vi "Three Button Dialog CORE - JKI.vi"(4 "Allow user to close window? (TRUE)":bool=TRUE, 5 "Justify Message (Left)":enum16{"Left", "Center", "Right"}(ring), 6 "Keyboard Shortcuts (Left is <Enter>)":T2={"Left Button Key Shortcut"={"Control"=FALSE, "Shift"=FALSE, "Key"="<Enter>"}, "Center Button Key Shortcut"={"Control"=FALSE, "Shift"=FALSE, "Key"=""}, "Right Button Key Shortcut"={"Control"=FALSE, "Shift"=FALSE, "Key"=""}}, 7 "Window Title (\"\")":string, 8 "Right Button Text (\"Cancel\")":string="Cancel", 9 "Center Button Text (\"No\")":string="No", 10 "Left Button Text (\"Yes\")":string="Yes", 11 "message":string) -> (3 "Which Button?":T1(ring)=enum."Center Button")   [LabVIEW 2013]
doc: "This is an example to show how someone can use the JKI State Machine. We show how you can refactor existing code. We have taken the 3 button dialog that ships with the base version of LabVIEW and upgraded it to use the JKI State Machine template.\n<B>The original VI is located at: <vi.lib>\\Utility\\error.llb\\Three Button Dialog CORE.vi</B>\n\nFor instructions on how to use the JKI State Machine, examples and video tutorials, visit:\nhttp://jkisoft.com/state-machine/\n\nJKI State Machine™ Example Code\nhttp://jkisoft.com/state-machine/\nCopyright (C) 2005-2008, JKI <info@jkisoft.com>\nALL RIGHTS RESERVED"
panel:
  in  "Right Button":bool
  in  "Center Button":bool
  in  "Left Button":bool
  out "C-Message":string
  in  "OK":string="OK"
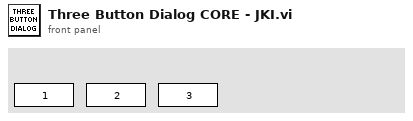
[diagram p1: front panel]
types:
  T1 = enum16{"Left Button", "Center Button", "Right Button", "Window Close"}
  T2 = cluster{"Left Button Key Shortcut":cluster{"Control":bool, "Shift":bool, "Key":string}, "Center Button Key Shortcut":cluster{"Control":bool, "Shift":bool, "Key":string}, "Right Button Key Shortcut":cluster{"Control":bool, "Shift":bool, "Key":string}}
  T3 = enum32{"invalid app kind", "Development System", "Run Time System", "Student Edition", "Embedded LabVIEW", "Evaluation", "Custom"}
  T4 = enum32{"Invalid", "Standard", "Closed", "Hidden", "Minimized", "Maximized"}
  T5 = cluster{"left":i16, "top":i16, "right":i16, "bottom":i16}
  T6 = cluster{"Core":cluster{"Current VI Reference":refnum<vi>, "Close Panel on Exit?":bool}, "Justify Message (Left)":enum16{"Left", "Center", "Right"}, "Allow user to close window? (TRUE)":bool, "Keyboard Shortcuts (Left is <Enter>)":cluster{"Left Button Key Shortcut":cluster{"Control":bool, "Shift":bool, "Key":string}, "Center Button Key Shortcut":cluster{"Control":bool, "Shift":bool, "Key":string}, "Right Button Key Shortcut":cluster{"Control":bool, "Shift":bool, "Key":string}}, "Left Button Text (\"Yes\")":string, "Center Button Text (\"No\")":string, "Right Button Text (\"Cancel\")":string, "message":string, "OK":string, "Left Visible?":bool, "Center Visible?":bool, "Right Visible?":bool, "C Message Height":u32, "minimum width for message":i32, "mimimum window width":i32, "minimum window width for buttons":i32, "Left Button Position:Left":i32, "grid spacing":i32, "grid spacing X2":i32, "window center":i32, "Window Title (\"\")":string, "Original FP.Title":string, "Which Button?":enum16{"Left Button", "Center Button", "Right Button", "Window Close"}}
  T7 = cluster{"Current VI Reference":refnum<vi>, "Close Panel on Exit?":bool}
  T8 = cluster{"Control":bool, "Shift":bool, "Key":string}
  T9 = cluster{bool, "Control":bool, "Shift":bool, "Key":string}
  T10 = typedef "LVRectTypeDef.ctl" = cluster{"Left":i16, "Top":i16, "Right":i16, "Bottom":i16}
  T11 = typedef "LVPointTypeDef.ctl" = cluster{"Horizontal":i16, "Vertical":i16}
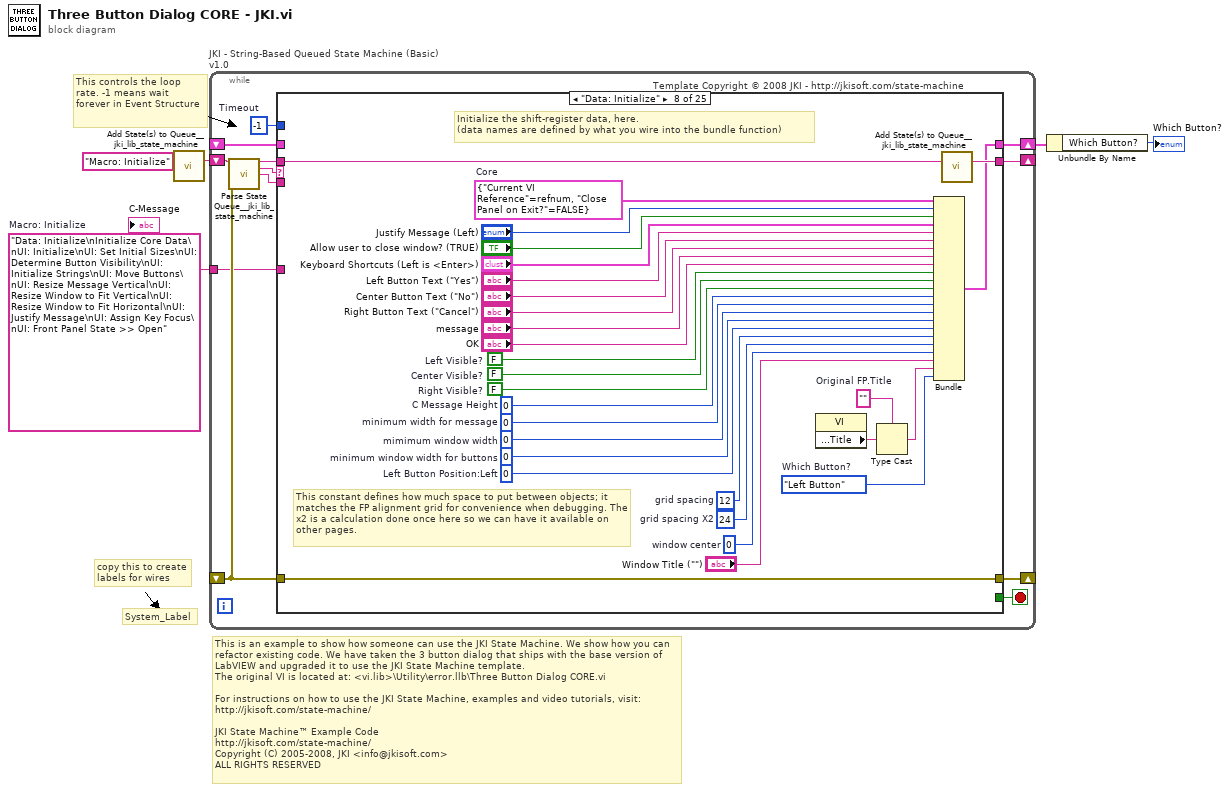
[diagram p0: block diagram]
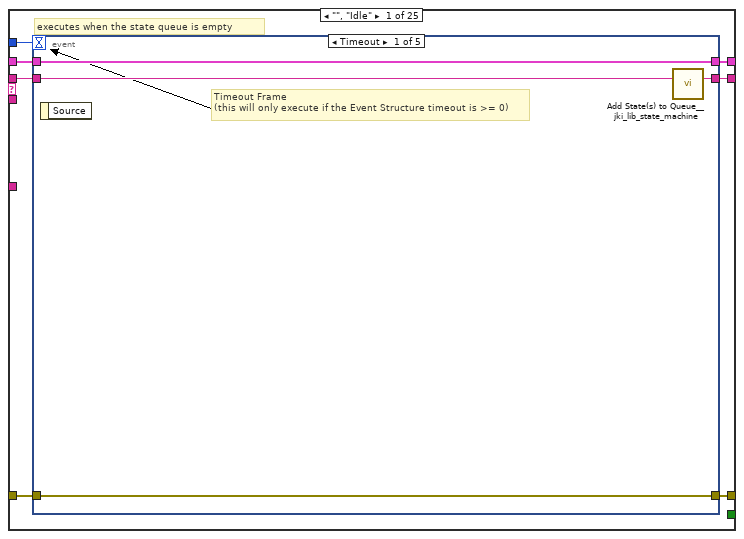
[diagram p2: hidden frame]
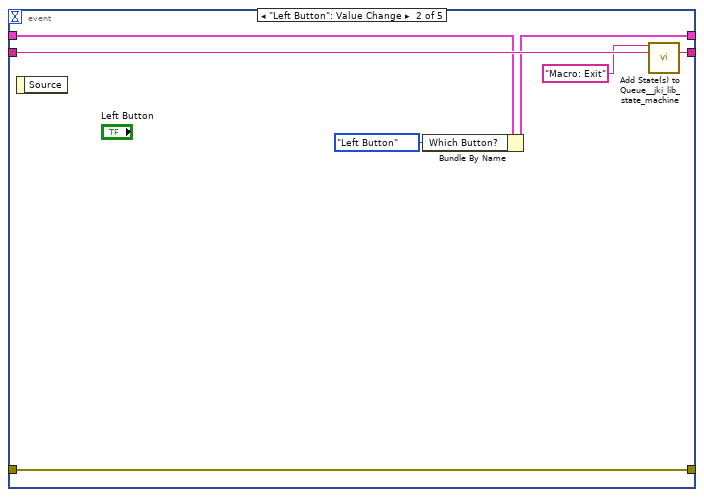
[diagram p3: hidden frame]
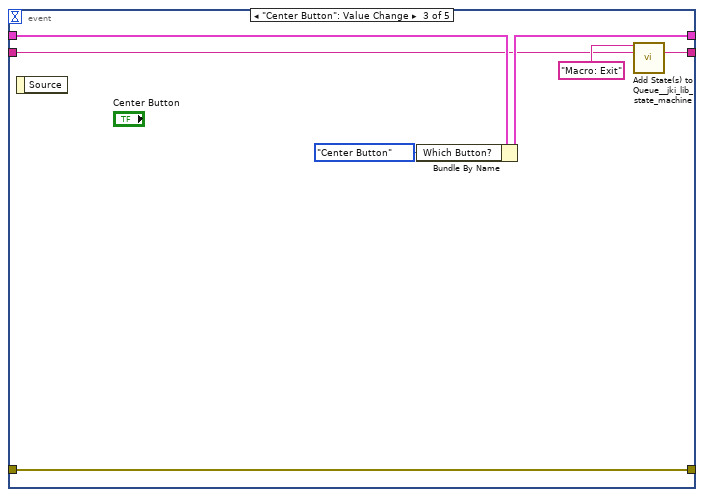
[diagram p4: hidden frame]
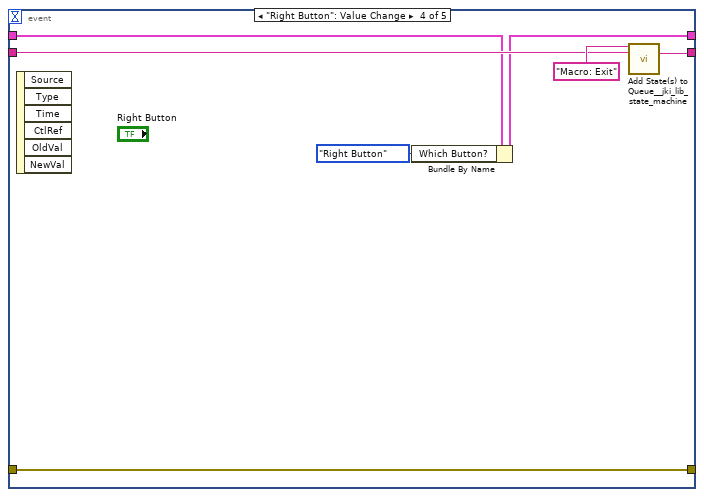
[diagram p5: hidden frame]
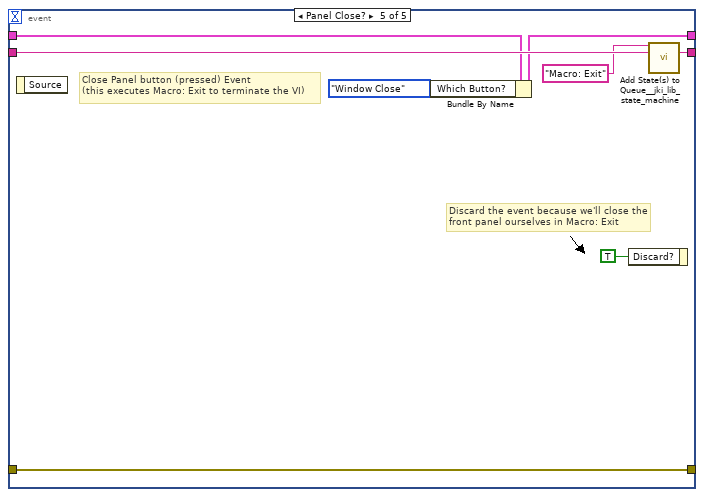
[diagram p6: hidden frame]
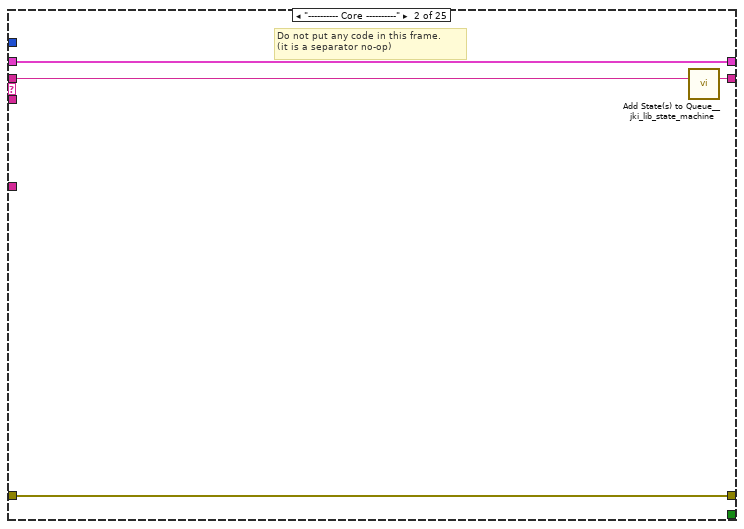
[diagram p7: hidden frame]
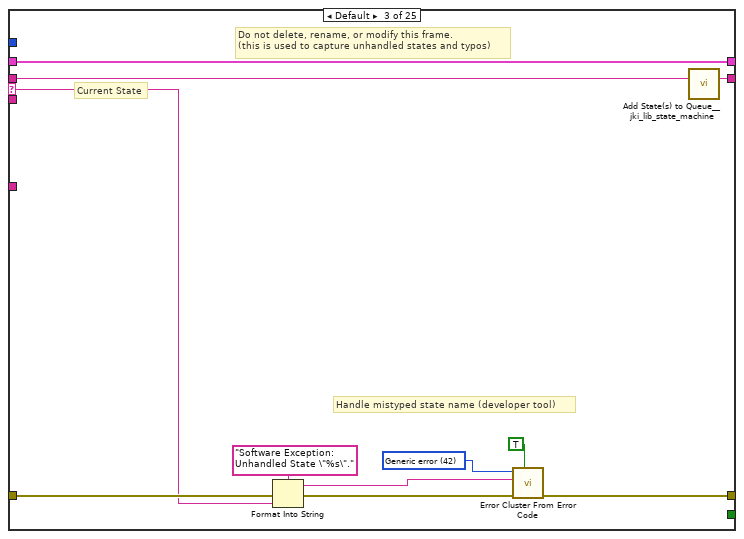
[diagram p8: hidden frame]
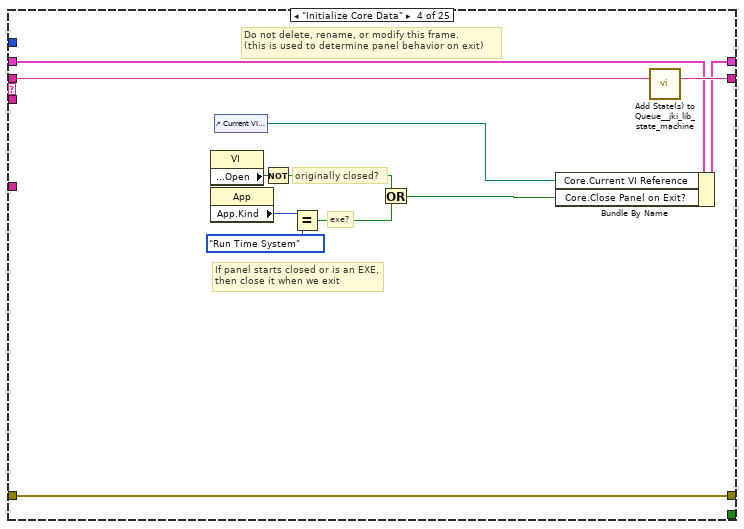
[diagram p9: hidden frame]
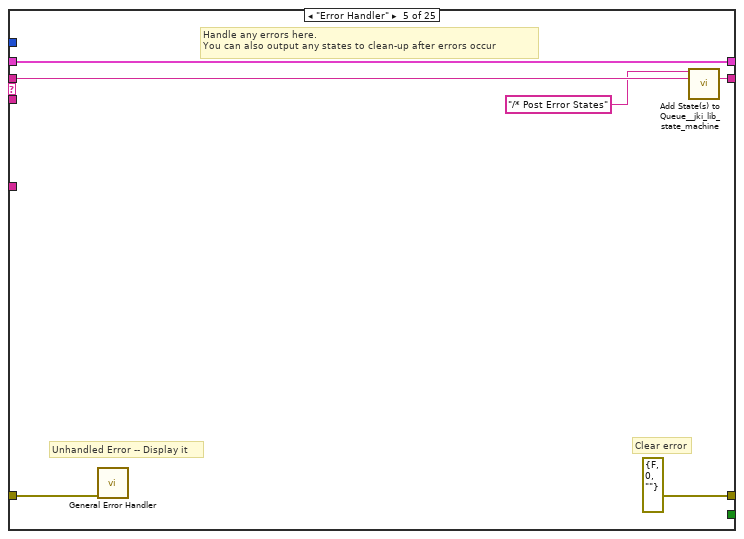
[diagram p10: hidden frame]
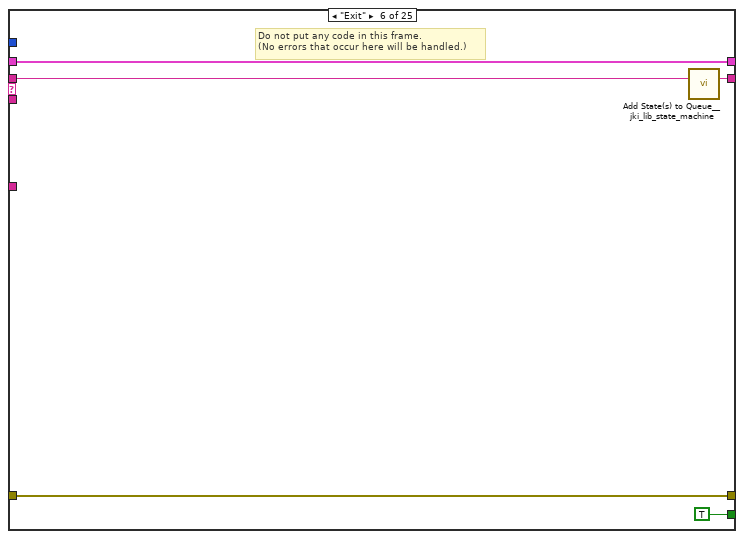
[diagram p11: hidden frame]
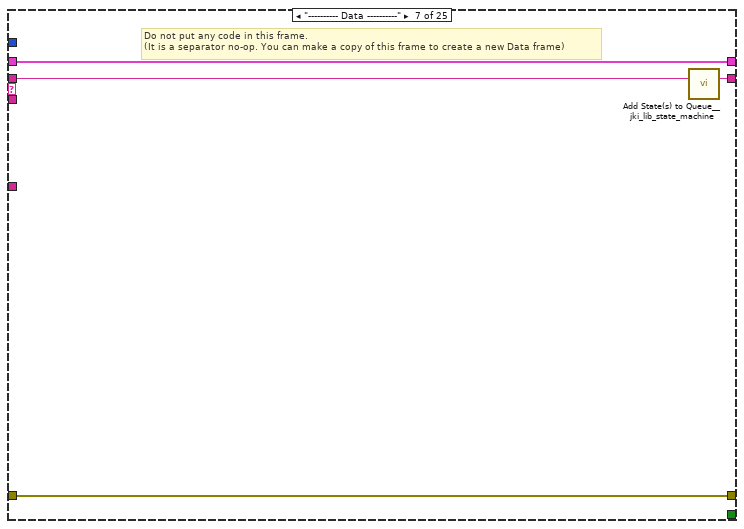
[diagram p12: hidden frame]
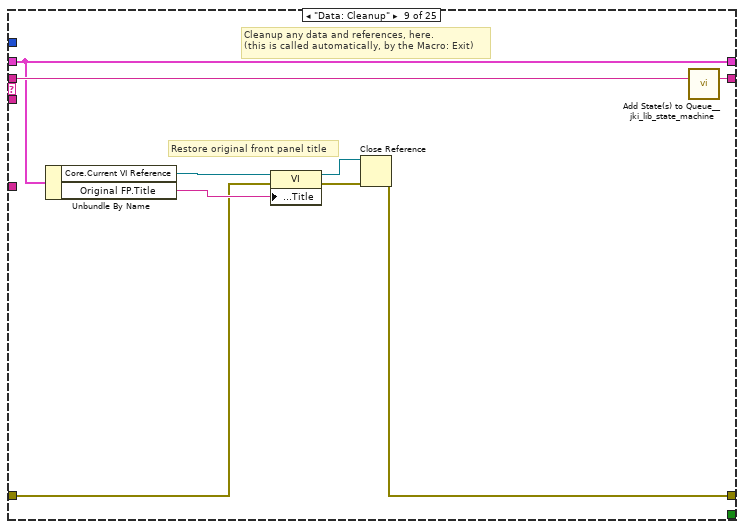
[diagram p13: hidden frame]
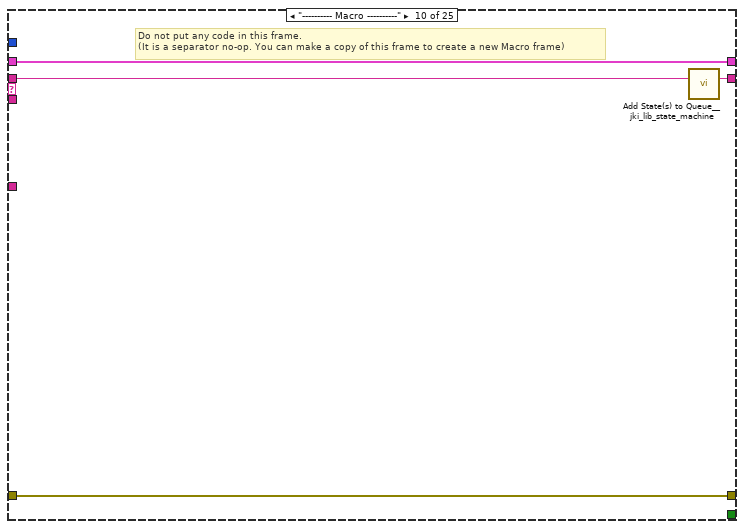
[diagram p14: hidden frame]
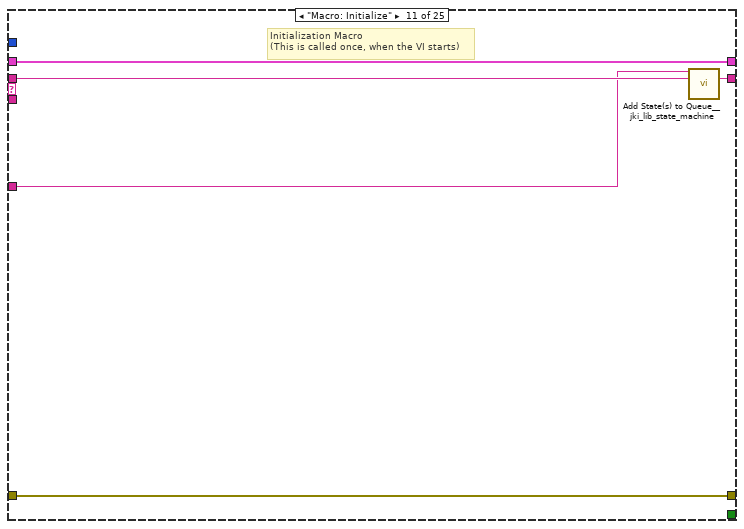
[diagram p15: hidden frame]
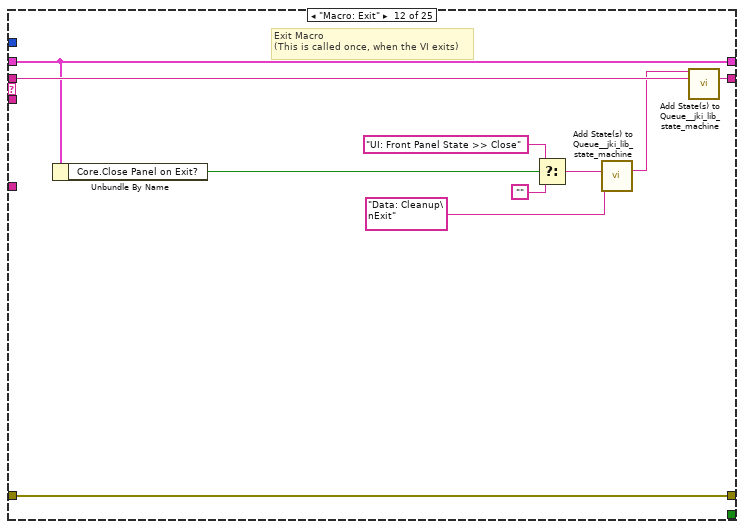
[diagram p16: hidden frame]
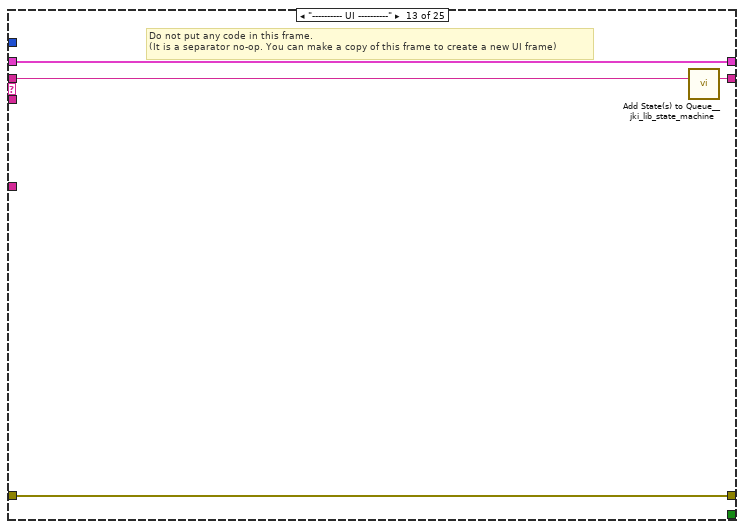
[diagram p17: hidden frame]
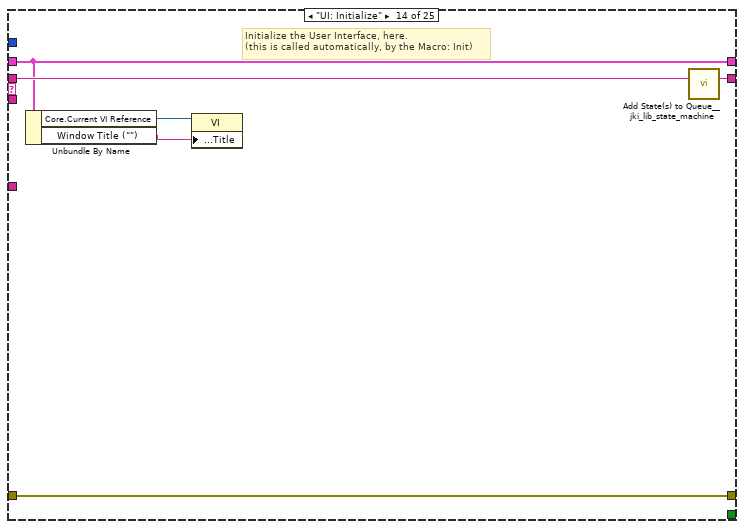
[diagram p18: hidden frame]
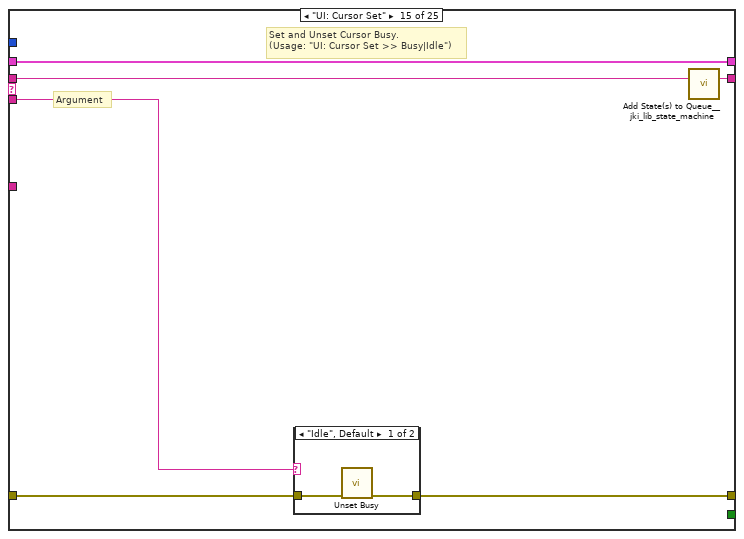
[diagram p19: hidden frame]
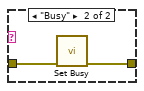
[diagram p20: hidden frame]
diagram:
  w1 = "Data: Initialize\nInitialize Core Data\nUI: Initialize\nUI: Set Initial Sizes\nUI: Determine Button Visibility\nUI: Initialize Strings\nUI: Move Buttons\nUI: Resize Message Vertical\nUI: Resize Window to Fit Vertical\nUI: Resize Window to Fit Horizontal\nUI: Justify Message\nUI: Assign Key Focus\nUI: Front Panel State >> Open"  # Macro: Initialize
  # "This is an example to show how someone can use the JKI State Machine. We show how you can refactor existing code. We have taken the 3 button dialog that ships with the base version of LabVIEW and upgraded it to use the JKI State Machine template.\nThe original VI is located at: <vi.lib>\\Utility\\error.llb\\Three Button Dialog CORE.vi\n\nFor instructions on how to use the JKI State Machine, examples and video tutorials, visit:\nhttp://jkisoft.com/state-machine/\n\nJKI State Machine™ Example Code\nhttp://jkisoft.com/state-machine/\nCopyright (C) 2005-2008, JKI <info@jkisoft.com>\nALL RIGHTS RESERVED"
  # "copy this to create labels for wires"
  # "This controls the loop rate. -1 means wait forever in Event Structure"
  # "System_Label"
  n1 = call <vilib>:"Add State(s) to Queue__jki_lib_state_machine.vi"("State(s) in (\"\")"="Macro: Initialize") -> ("States Out"=w4:string)  [unwired: 14 in]
  n2 = while "JKI - String-Based Queued State Machine (Basic) v1.0" {
    shift-right: [w10] -> w3
    shift-left: _ -> [w9]
    shift-right: [w13] -> _
    shift-left: _ -> [w7]
    shift-right: [w12] -> _
    shift-left: w4 -> [w14]
    tunnel: w1 -> [w6]
    stop <- w11 stop-if-true
    w8 = -1  # Timeout
    # "Template Copyright © 2008 JKI - http://jkisoft.com/state-machine"
    n3 = call <vilib>:"Parse State Queue__jki_lib_state_machine.vi"("State Queue"=w14, "Error In (no error)"=w7) -> ("Remaining States"=w16:string, "Current State"=w17:string, "Arguments"=w15:string)  [unwired: 11 in]
    n4 = case shown="\"Data: Initialize\"" w17 {
      selector: w17 -> [_ _ w62 _ _ _ _ _ _ _ _ _ _ _ _ _ _ _ _ _ _ _ _ _ _]
      tunnel: w16 -> [w24 w61 w66 w84 w90 w95 w99 w128 w137 w141 w146 w156 w160 w166 w172 w185 w231 w248 w283 w329 w364 w393 w417 w459 w496]
      tunnel: w15 -> [_ _ _ _ _ _ _ _ _ _ _ _ _ _ w167 w181 _ _ _ _ _ _ _ _ _]
      tunnel: w9 -> [w22 w58 w64 w75 w87 w93 w96 _ w134 w138 w143 w153 w157 w163 w170 w182 w218 w238 w256 w304 w353 w373 w396 w448 w493]
      tunnel: [w21 w59 w68 w81 errorcluster {"status"=FALSE, "code"=0, "source"=""} ("error out") w92 w97 w125 w135 w139 w144 w154 w158 w164 w168 w183 w213 w246 w281 w327 w362 w391 w415 w457 w494] -> w13
      tunnel: w7 -> [w20 w59 w67 w81 w86 w92 w97 w125 w129 w139 w144 w154 w158 w164 w169 w177 w210 w246 w281 w327 w362 w391 w415 w457 w494]
      tunnel: [w23 w60 w65 w83 w89 w94 w98 w127 w136 w140 w145 w155 w159 w165 w171 w184 w230 w247 w282 w328 w363 w392 w416 w458 w495] -> w12
      tunnel: [_ _ _ _ _ TRUE _ _ _ _ _ _ _ _ _ _ _ _ _ _ _ _ _ _ _] -> w11
      tunnel: [w19 w58 w64 w82 w87 w93 w96 w126 w134 w138 w143 w153 w157 w163 w170 w182 w218 w237 w255 w303 w353 w373 w397 w448 w493] -> w10
      tunnel: w8 -> [w18 _ _ _ _ _ _ _ _ _ _ _ _ _ _ _ _ _ _ _ _ _ _ _ _]
      tunnel: w6 -> [_ _ _ _ _ _ _ _ _ _ w142 _ _ _ _ _ _ _ _ _ _ _ _ _ _]
      frame "", "Idle" {
        # "executes when the state queue is empty"
        n5 = event shown="[0] Timeout" {
          selector: _ -> [_ _ _ _ _]
          dyn-events: _ -> [_ _ _ _ _]
          timeout: w18 -> [_ _ _ _ _]
          tunnel: w24 -> [w28 w35 w37 w47 w57]
          tunnel: [w27 w34 w39 w46 w56] -> w23
          tunnel: w22 -> [w25 w31 w41 w44 w52]
          tunnel: [w26 w33 w36 w43 w55] -> w21
          tunnel: w20 -> [w26 w33 w36 w43 w55]
          tunnel: [w25 w30 w40 w45 w51] -> w19
          event Timeout {
            # "Timeout Frame\n(this will only execute if the Event Structure timeout is >= 0)"
            n6 = event-data() -> ()  [unwired: 1 in, 1 out]
            n7 = call <vilib>:"Add State(s) to Queue__jki_lib_state_machine.vi"("State(s) in (\"\")"=w28) -> ("States Out"=w27:string)  [unwired: 14 in]
          }
          event "Left Button": Value Change {
            n8 = event-data() -> ()  [unwired: 1 in, 1 out]
            n9 = Bundle By Name(cluster=w31, "Which Button?"=T1."Left Button") -> (w30:T6)
            n10 = call <vilib>:"Add State(s) to Queue__jki_lib_state_machine.vi"("State(s) in Front (\"\")"="Macro: Exit", "State(s) in (\"\")"=w35) -> ("States Out"=w34:string)  [unwired: 13 in]
          }
          event "Center Button": Value Change {
            n11 = event-data() -> ()  [unwired: 1 in, 1 out]
            n12 = Bundle By Name(cluster=w41, "Which Button?"=T1."Center Button") -> (w40:T6)
            n13 = call <vilib>:"Add State(s) to Queue__jki_lib_state_machine.vi"("State(s) in Front (\"\")"="Macro: Exit", "State(s) in (\"\")"=w37) -> ("States Out"=w39:string)  [unwired: 13 in]
          }
          event "Right Button": Value Change {
            n14 = event-data() -> ()  [unwired: 1 in, 6 out]
            n15 = Bundle By Name(cluster=w44, "Which Button?"=T1."Right Button") -> (w45:T6)
            n16 = call <vilib>:"Add State(s) to Queue__jki_lib_state_machine.vi"("State(s) in Front (\"\")"="Macro: Exit", "State(s) in (\"\")"=w47) -> ("States Out"=w46:string)  [unwired: 13 in]
          }
          event Panel Close? {
            # "Discard the event because we'll close the front panel ourselves in Macro: Exit"
            # "Close Panel button (pressed) Event\n(this executes Macro: Exit to terminate the VI)"
            n17 = event-data() -> ()  [unwired: 1 in, 1 out]
            n18 = Bundle By Name(cluster=w52, "Which Button?"=T1."Window Close") -> (w51:T6)
            n19 = event-data("Discard?"=TRUE) -> ()  [unwired: 1 in, 1 out]
            n20 = call <vilib>:"Add State(s) to Queue__jki_lib_state_machine.vi"("State(s) in Front (\"\")"="Macro: Exit", "State(s) in (\"\")"=w57) -> ("States Out"=w56:string)  [unwired: 13 in]
          }
        }
      }
      frame "---------- Core ----------" {
        # "Do not put any code in this frame.\n(it is a separator no-op)"
        n21 = call <vilib>:"Add State(s) to Queue__jki_lib_state_machine.vi"("State(s) in (\"\")"=w61) -> ("States Out"=w60:string)  [unwired: 14 in]
      }
      frame Default {
        w71 = 42 items=["No error", "Argument error", "Memory is full", "Out of zone", "End of file", "File already open", "Generic file I/O error", "File not found", "File permission error", "Disk is full", "Duplicate path", "Too many files open", "System feature not enabled", "Resource file not found", "Cannot add resource", "Resource not found", "Image not found", "Image memory error", "Pen does not exist", "Config type invalid", "Config token not found", "Config parse error", "Config memory error", "Bad external code format", "Bad external code offset", "External code not present", "Null window", "Destroy window error", "Null menu", "Print aborted", "Bad print record", "Print driver error", "Windows error during printing", "Memory error during printing", "Print dialog error", "Generic print error", "Invalid device refnum", "Device not found", "Device parameter error", "Device unit error", "Cannot open device", "Device call aborted", "Generic error", "Cancelled by user", "Object ID too low", "Object ID too high", "Object not in heap", "Unknown heap", "Unknown object (invalid DefProc)", "Unknown object (DefProc not in table)", "Message out of range", "Invalid (null) method", "Unknown message", "Manager call not supported", "Bad address", "Network operation in progress", "Network operation timed out", "Connection is busy", "Network attribute not supported", "Network error", "Address in use", "System out of memory", "Connection aborted", "Connection refused", "Not connected", "Already connected", "Connection closed", "Initialization error (interapplication manager)", "Bad occurrence", "Wait on unbound occurrence handler", "Occurrence queue overflow", "Datalog type conflict", "Unused", "Unrecognized type (interapplication manager)", "Memory corrupt", "Failed to make temporary DLL", "Old CIN version", "Drag socket not found", "Failed to load drop-object", "Failed to register OLE object", "Failed to release OLE object", "Format specifier type mismatch", "Unknown format specifier", "Too few format specifiers", "Too many format specifiers", "Scan failed", "Newer CIN version", "Error converting to variant", "Runtime menu error", "Password tampered", "Variant attribute not found", "Incompatible variant data type", "Event data is not available", "Event Store is not present", "Occurrence is not found", "Event Queue is not created", "Event info is not available", "Refnum passed is NULL", "Error retrieving Class GUID", "Error retrieving CoClass GUID", "Error retrieving TypeLib GUID.", "Bad built application magic bytes.", "Specific driver is different from the specific driver associated with the Logical Name.", "There is no session opened to the class driver.", "Max Error", "MAX - Error with config objects", "MAX - Error loading configuration", "MAX - Group not supported"]
        # "Current State"
        # "Do not delete, rename, or modify this frame.\n(this is used to capture unhandled states and typos)"
        # "Handle mistyped state name (developer tool)"
        n22 = Format Into String(format string="Software Exception: Unhandled State \"%s\"." ("message"), error in=w67, w62) -> (resulting string=w70:string, error out=w69:errorcluster)  [unwired: 1 in]
        n23 = call <vilib>:"Error Cluster From Error Code.vi"("show call chain? (False)"=TRUE, "error in (no error)"=w69, "error message (\"\")"=w70, "error code (0)"=w71) -> ("error out"=w68:errorcluster)  [unwired: 5 in]
        n24 = call <vilib>:"Add State(s) to Queue__jki_lib_state_machine.vi"("State(s) in (\"\")"=w66) -> ("States Out"=w65:string)  [unwired: 14 in]
      }
      frame "Initialize Core Data" {
        # "Do not delete, rename, or modify this frame.\n(this is used to determine panel behavior on exit)"
        # "originally closed?"
        # "exe?"
        # "If panel starts closed or is an EXE, then close it when we exit"
        n25 = property class="VI"() -> ("Front Panel.Open"=w80:bool)  [unwired: 2 in, 2 out]
        n26 = property class="App"() -> ("App.Kind"=w79:T3)  [unwired: 2 in, 2 out]
        n27 = control-ref of="Current VI Reference"() -> (w73:refnum<vi>)
        n28 = Not(x=w80) -> (.not. x?=w77:bool)
        n29 = Equal?(x=w79, y=T3."Run Time System" ("Application:Kind")) -> (x = y?=w76:bool)
        n30 = Or(x=w77, y=w76) -> (x .or. y?=w74:bool)
        n31 = Bundle By Name(cluster=w75, "Core.Current VI Reference"=w73, "Core.Close Panel on Exit?"=w74) -> (w82:T6)
        n32 = call <vilib>:"Add State(s) to Queue__jki_lib_state_machine.vi"("State(s) in (\"\")"=w84) -> ("States Out"=w83:string)  [unwired: 14 in]
      }
      frame "Error Handler" {
        # "Unhandled Error -- Display it"
        # "Handle any errors here.\nYou can also output any states to clean-up after errors occur"
        # "Clear error"
        n33 = call <vilib>:"General Error Handler.vi"("error in (no error)"=w86) -> ()  [unwired: 10 in, 5 out]
        n34 = call <vilib>:"Add State(s) to Queue__jki_lib_state_machine.vi"("State(s) in Front (\"\")"="/* Post Error States", "State(s) in (\"\")"=w90) -> ("States Out"=w89:string)  [unwired: 13 in]
      }
      frame "Exit" {
        # "Do not put any code in this frame.\n(No errors that occur here will be handled.)"
        n35 = call <vilib>:"Add State(s) to Queue__jki_lib_state_machine.vi"("State(s) in (\"\")"=w95) -> ("States Out"=w94:string)  [unwired: 14 in]
      }
      frame "---------- Data ----------" {
        # "Do not put any code in this frame.\n(It is a separator no-op. You can make a copy of this frame to create a new Data frame)"
        n36 = call <vilib>:"Add State(s) to Queue__jki_lib_state_machine.vi"("State(s) in (\"\")"=w99) -> ("States Out"=w98:string)  [unwired: 14 in]
      }
      frame "Data: Initialize" {
        w100 = T1."Left Button"  # Which Button?
        w105 = 0  # window center
        w106 = 24  # grid spacing X2
        w107 = 12  # grid spacing
        w108 = 0  # Left Button Position:Left
        w109 = 0  # minimum window width for buttons
        w110 = 0  # mimimum window width
        w111 = 0  # minimum width for message
        w112 = u32 0  # C Message Height
        w102 = ""  # Original FP.Title
        w124 = T7 {"Current VI Reference"=refnum, "Close Panel on Exit?"=FALSE}  # Core
        w113 = FALSE  # Right Visible?
        w114 = FALSE  # Center Visible?
        w115 = FALSE  # Left Visible?
        # "This constant defines how much space to put between objects; it matches the FP alignment grid for convenience when debugging. The x2 is a calculation done once here so we can have it available on other pages."
        # "Initialize the shift-register data, here.\n(data names are defined by what you wire into the bundle function)"
        n37 = property class="VI"() -> ("Front Panel Window:Title"=w103:string)  [unwired: 2 in, 2 out]
        n38 = Type Cast(type=w102, x=w103) -> (*(type *) &x=w101:string)
        n39 = Bundle("Core"=w124, "Justify Message (Left)"="Justify Message (Left)", "Allow user to close window? (TRUE)"="Allow user to close window? (TRUE)", "Keyboard Shortcuts (Left is <Enter>)"="Keyboard Shortcuts (Left is <Enter>)", "Left Button Text (\"Yes\")"="Left Button Text (\"Yes\")", "Center Button Text (\"No\")"="Center Button Text (\"No\")", "Right Button Text (\"Cancel\")"="Right Button Text (\"Cancel\")", "message"="message", "OK"="OK", "Left Visible?"=w115, "Center Visible?"=w114, "Right Visible?"=w113, "C Message Height"=w112, "minimum width for message"=w111, "mimimum window width"=w110, "minimum window width for buttons"=w109, "Left Button Position:Left"=w108, "grid spacing"=w107, "grid spacing X2"=w106, "window center"=w105, "Window Title (\"\")"="Window Title (\"\")", "Original FP.Title"=w101, "Which Button?"=w100) -> (w126:T6)  [unwired: 1 in]
        n40 = call <vilib>:"Add State(s) to Queue__jki_lib_state_machine.vi"("State(s) in (\"\")"=w128) -> ("States Out"=w127:string)  [unwired: 14 in]
      }
      frame "Data: Cleanup" {
        # "Restore original front panel title"
        # "Cleanup any data and references, here.\n(this is called automatically, by the Macro: Exit)"
        n41 = Unbundle By Name(w134) -> ("Core.Current VI Reference"=w132:refnum<vi>, "Original FP.Title"=w133:string)
        n42 = property class="VI"(reference=w132, error in=w129, "Front Panel Window:Title"=w133) -> (reference out=w131:refnum<vi>, error out=w130:errorcluster)
        n43 = Close Reference(reference=w131, error in (no error)=w130) -> (error out=w135:errorcluster)
        n44 = call <vilib>:"Add State(s) to Queue__jki_lib_state_machine.vi"("State(s) in (\"\")"=w137) -> ("States Out"=w136:string)  [unwired: 14 in]
      }
      frame "---------- Macro ----------" {
        # "Do not put any code in this frame.\n(It is a separator no-op. You can make a copy of this frame to create a new Macro frame)"
        n45 = call <vilib>:"Add State(s) to Queue__jki_lib_state_machine.vi"("State(s) in (\"\")"=w141) -> ("States Out"=w140:string)  [unwired: 14 in]
      }
      frame "Macro: Initialize" {
        # "Initialization Macro\n(This is called once, when the VI starts)"
        n46 = call <vilib>:"Add State(s) to Queue__jki_lib_state_machine.vi"("State(s) in Front (\"\")"=w142, "State(s) in (\"\")"=w146) -> ("States Out"=w145:string)  [unwired: 13 in]
      }
      frame "Macro: Exit" {
        # "Exit Macro\n(This is called once, when the VI exits)"
        n47 = Unbundle By Name(w153) -> ("Core.Close Panel on Exit?"=w152:bool)
        n48 = Select(t="UI: Front Panel State >> Close", s=w152, f="") -> (s? t:f=w149:string)
        n49 = call <vilib>:"Add State(s) to Queue__jki_lib_state_machine.vi"("State(s) in (\"\")"=w149, "State(s) at Back (\"\")"="Data: Cleanup\nExit") -> ("States Out"=w147:string)  [unwired: 13 in]
        n50 = call <vilib>:"Add State(s) to Queue__jki_lib_state_machine.vi"("State(s) in Front (\"\")"=w147, "State(s) in (\"\")"=w156) -> ("States Out"=w155:string)  [unwired: 13 in]
      }
      frame "---------- UI ----------" {
        # "Do not put any code in this frame.\n(It is a separator no-op. You can make a copy of this frame to create a new UI frame)"
        n51 = call <vilib>:"Add State(s) to Queue__jki_lib_state_machine.vi"("State(s) in (\"\")"=w160) -> ("States Out"=w159:string)  [unwired: 14 in]
      }
      frame "UI: Initialize" {
        # "Initialize the User Interface, here.\n(this is called automatically, by the Macro: Init)"
        n52 = Unbundle By Name(w163) -> ("Core.Current VI Reference"=w161:refnum<vi>, "Window Title (\"\")"=w162:string)
        n53 = property class="VI"(reference=w161, "Front Panel Window:Title"=w162) -> ()  [unwired: 1 in, 2 out]
        n54 = call <vilib>:"Add State(s) to Queue__jki_lib_state_machine.vi"("State(s) in (\"\")"=w166) -> ("States Out"=w165:string)  [unwired: 14 in]
      }
      frame "UI: Cursor Set" {
        # "Argument"
        # "Set and Unset Cursor Busy.\n(Usage: \"UI: Cursor Set >> Busy|Idle\")"
        n55 = case shown="\"Idle\", Default" w167 {
          tunnel: w169 -> [w174 w176]
          tunnel: [w173 w175] -> w168
          frame "Idle", Default {
            n56 = call <vilib>:"Unset Busy.vi"("error in (no error)"=w174) -> ("error out"=w173:errorcluster)  [unwired: 10 in]
          }
          frame "Busy" {
            n57 = call <vilib>:"Set Busy.vi"("error in (no error)"=w176) -> ("error out"=w175:errorcluster)  [unwired: 9 in, 1 out]
          }
        }
        n58 = call <vilib>:"Add State(s) to Queue__jki_lib_state_machine.vi"("State(s) in (\"\")"=w172) -> ("States Out"=w171:string)  [unwired: 14 in]
      }
      frame "UI: Front Panel State" {
        # "Argument"
        # "Set Front Panel Open or Closed\n(Usage: \"UI: Front Panel State >> Open|Close\")"
        n59 = Unbundle By Name(w182) -> ("Core.Current VI Reference"=w180:refnum<vi>)
        n60 = invoke class="VI" method="FP.Center"(reference=w180, error in=w177) -> (reference out=w179:refnum<vi>, error out=w178:errorcluster)  [unwired: 1 in, 1 out]
        n61 = case shown="\"Open\", Default" w181 {
          tunnel: w178 -> [w189 w202]
          tunnel: [w191 w203] -> w183
          tunnel: w179 -> [w190 w200]
          frame "Open", Default {
            n62 = property class="VI"(reference=w190, error in=w189) -> (reference out=w187:refnum<vi>, error out=w188:errorcluster, "Front Panel.Open"=w186:bool)
            n63 = case shown="False" w186 {
              tunnel: [w194 w197] -> w191
              tunnel: w188 -> [w193 w197]
              tunnel: w187 -> [w192 _]
              frame False {
                n64 = invoke class="VI" method="FP.Open"(reference=w192, error in=w193, "Activate"=TRUE, "State"=T4."Standard") -> (error out=w194:errorcluster)  [unwired: 1 in, 4 out]
              }
              frame True {
              }
            }
          }
          frame "Close" {
            n65 = property class="VI"(reference=w200, error in=w202) -> (reference out=w199:refnum<vi>, error out=w201:errorcluster, "Front Panel.Open"=w198:bool)
            n66 = case shown="True" w198 {
              tunnel: [w204 w207] -> w203
              tunnel: w201 -> [w204 w206]
              tunnel: w199 -> [_ w205]
              frame False {
              }
              frame True {
                n67 = invoke class="VI" method="FP.Close"(reference=w205, error in=w206) -> (error out=w207:errorcluster)  [unwired: 1 in, 2 out]
              }
            }
          }
        }
        n68 = call <vilib>:"Add State(s) to Queue__jki_lib_state_machine.vi"("State(s) in (\"\")"=w185) -> ("States Out"=w184:string)  [unwired: 14 in]
      }
      frame "UI: Set Initial Sizes" {
        w229 = string[] [" ", " ", " ", " "] ("Strings [4]")
        w228 = cluster{"Width":u32, "Height":u32} {"Width"=60, "Height"=24} ("Button Size")
        # "This sets up initial sizes and viewing rectangles\nfor the VI and its controls. This initialization\nsimplifies the task of moving controls to their\ncorrect dynamic locations. This also gives us our\nminimum bounds for the window."
        n69 = Unbundle By Name(w218) -> ("Justify Message (Left)"=w217:enum16{"Left", "Center", "Right"}, "Allow user to close window? (TRUE)"=w212:bool, "Core.Current VI Reference"=w209:refnum<vi>)
        n70 = property class="VI"(reference=w209, error in=w210, "Front Panel Window:Closeable"=w212) -> (reference out=w208:refnum<vi>, error out=w211:errorcluster)
        n71 = property class="VI"(reference=w208, error in=w211, "Front Panel Window:Panel Bounds"=T5 {"left"=338, "top"=316, "right"=686, "bottom"=392} ("Front Panel.PanelBounds")) -> (error out=w221:errorcluster)  [unwired: 1 out]
        n72 = property on="Pane" class="Pane"(error in=w221, "Origin"=cluster{"Horizontal":i16, "Vertical":i16} {"Horizontal"=-191, "Vertical"=109} ("Front Panel.Origin")) -> (error out=w220:errorcluster)  [unwired: 1 in, 1 out]
        n73 = property on="C-Message" class="Str"(error in=w220, "Text.Justification"=w217, "Value"="") -> (error out=w224:errorcluster)  [unwired: 1 in, 1 out]
        n74 = invoke on="C-Message" class="Str" method="Size to Text"(error in=w224) -> (error out=w216:errorcluster)  [unwired: 2 in, 2 out]
        n75 = property on="Left Button" class="Bool"(error in=w216, "Strings [4]"=w229, "Button Size"=w228, "Position"=cluster{"Left":i32, "Top":i32} {"Left"=-180, "Top"=156}) -> (error out=w215:errorcluster)  [unwired: 1 in, 1 out]
        n76 = property on="Center Button" class="Bool"(error in=w215, "Strings [4]"=w229, "Button Size"=w228, "Position"=cluster{"Left":i32, "Top":i32} {"Left"=-48, "Top"=156}) -> (error out=w214:errorcluster)  [unwired: 1 in, 1 out]
        n77 = property on="Right Button" class="Bool"(error in=w214, "Strings [4]"=w229, "Button Size"=w228, "Position"=cluster{"Left":i32, "Top":i32} {"Left"=84, "Top"=156}) -> (error out=w213:errorcluster)  [unwired: 1 in, 1 out]
        n78 = call <vilib>:"Add State(s) to Queue__jki_lib_state_machine.vi"("State(s) in (\"\")"=w231) -> ("States Out"=w230:string)  [unwired: 14 in]
      }
      frame "UI: Determine Button Visibility" {
        # "If left center and right is empty then center button =ok"
        n79 = Unbundle By Name(w238) -> ("OK"=w236:string, "Left Button Text (\"Yes\")"=w241:string, "Center Button Text (\"No\")"=w240:string, "Right Button Text (\"Cancel\")"=w239:string)
        n80 = Empty String/Path?(string/path=w241) -> (empty?=w245:bool)
        n81 = Empty String/Path?(string/path=w240) -> (empty?=w243:bool)
        n82 = Empty String/Path?(string/path=w239) -> (empty?=w242:bool)
        n83 = Not(x=w245) -> (.not. x?=w234:bool)
        n84 = Not(x=w242) -> (.not. x?=w232:bool)
        n85 = Compound Arithmetic op=AND(w245, w242, w243) -> (w244:bool)
        n86 = case shown="False" w244 {
          tunnel: w243 -> [w251 _]
          tunnel: [w250 TRUE] -> w233
          tunnel: w240 -> [w249 _]
          tunnel: [w249 w252] -> w235
          tunnel: w236 -> [_ w252]
          frame False {
            n87 = Not(x=w251) -> (.not. x?=w250:bool)
          }
          frame True {
          }
        }
        n88 = Bundle By Name(cluster=w238, "Center Button Text (\"No\")"=w235, "Left Visible?"=w234, "Center Visible?"=w233, "Right Visible?"=w232) -> (w237:T6)
        n89 = property on="Left Button" class="Bool"("Visible"=w234) -> ()  [unwired: 2 in, 2 out]
        n90 = property on="Center Button" class="Bool"("Visible"=w233) -> ()  [unwired: 2 in, 2 out]
        n91 = property on="Right Button" class="Bool"("Visible"=w232) -> ()  [unwired: 2 in, 2 out]
        n92 = call <vilib>:"Add State(s) to Queue__jki_lib_state_machine.vi"("State(s) in (\"\")"=w248) -> ("States Out"=w247:string)  [unwired: 14 in]
      }
      frame "UI: Initialize Strings" {
        w266 = FALSE
        # "Initialize all of our strings from our inputs."
        n93 = Unbundle By Name(w256) -> ("message"=w263:string)
        n94 = Unbundle By Name(w256) -> ("Keyboard Shortcuts (Left is <Enter>).Left Button Key Shortcut"=w279:T8, "Keyboard Shortcuts (Left is <Enter>).Center Button Key Shortcut"=w271:T8, "Keyboard Shortcuts (Left is <Enter>).Right Button Key Shortcut"=w265:T8)
        n95 = Unbundle By Name(w256) -> ("Right Button Text (\"Cancel\")"=w258:string, "Right Visible?"=w257:bool)
        n96 = Unbundle By Name(w256) -> ("Center Button Text (\"No\")"=w261:string, "Center Visible?"=w259:bool)
        n97 = Unbundle By Name(w256) -> ("Left Button Text (\"Yes\")"=w262:string, "Left Visible?"=w260:bool)
        n98 = flat-sequence {
          tunnel: [w284] -> w280
          tunnel: w280 -> [w288]
          tunnel: w263 -> [w289]
          tunnel: [w288] -> w254
          frame #0 {
            w287 = "M#,\"jqAW?><"  # One line of text
            n99 = property on="C-Message" class="Str"("Value"=w287) -> (error out=w285:errorcluster)  [unwired: 2 in, 1 out]
            n100 = invoke on="C-Message" class="Str" method="Size to Text"(error in=w285) -> (error out=w286:errorcluster)  [unwired: 2 in, 2 out]
            n101 = property on="C-Message" class="Str"(error in=w286) -> ("Height"=w284:u32)  [unwired: 1 in, 2 out]
          }
          frame #1 {
            n102 = property on="C-Message" class="Str"("Value"=w289) -> ()  [unwired: 2 in, 2 out]
          }
          frame #2 {
            n103 = local write "message"("") -> ()
          }
        }
        n104 = Unbundle(w279) -> ("Control"=w278:bool, "Shift"=w277:bool, "Key"=w276:string)
        n105 = Unbundle(w271) -> ("Control"=w274:bool, "Shift"=w273:bool, "Key"=w272:string)
        n106 = Unbundle(w265) -> ("Control"=w269:bool, "Shift"=w268:bool, "Key"=w267:string)
        n107 = Bundle(w266, "Control"=w269, "Shift"=w268, "Key"=w267) -> (w264:T9)  [unwired: 1 in]
        n108 = Bundle(w266, "Control"=w278, "Shift"=w277, "Key"=w276) -> (w275:T9)  [unwired: 1 in]
        n109 = Bundle(w266, "Control"=w274, "Shift"=w273, "Key"=w272) -> (w270:T9)  [unwired: 1 in]
        n110 = case shown="True" w259 {
          tunnel: w270 -> [_ w296]
          tunnel: w261 -> [_ w295]
          frame False {
          }
          frame True {
            n111 = Initialize Array(w295, 4 ("dimension size")) -> (w298:string[])
            n112 = property on="Center Button" class="Bool"("Strings [4]"=w298, "ToggleKeyBind"=w296) -> ()  [unwired: 2 in, 2 out]
          }
        }
        n113 = case shown="True" w260 {
          tunnel: w262 -> [_ w300]
          tunnel: w275 -> [_ w299]
          frame False {
          }
          frame True {
            n114 = Initialize Array(w300, 4 ("dimension size")) -> (w302:string[])
            n115 = property on="Left Button" class="Bool"("Strings [4]"=w302, "ToggleKeyBind"=w299) -> ()  [unwired: 2 in, 2 out]
          }
        }
        n116 = case shown="True" w257 {
          tunnel: w264 -> [_ w292]
          tunnel: w258 -> [_ w291]
          frame False {
          }
          frame True {
            n117 = Initialize Array(w291, 4 ("dimension size")) -> (w294:string[])
            n118 = property on="Right Button" class="Bool"("Strings [4]"=w294, "ToggleKeyBind"=w292) -> ()  [unwired: 2 in, 2 out]
          }
        }
        n119 = Bundle By Name(cluster=w256, "C Message Height"=w254) -> (w255:T6)
        n120 = call <vilib>:"Add State(s) to Queue__jki_lib_state_machine.vi"("State(s) in (\"\")"=w283) -> ("States Out"=w282:string)  [unwired: 14 in]
      }
      frame "UI: Move Buttons" {
        # "position of left edge"
        # "In the previous page, we set new bool text strings for all our buttons. This causes the buttons to resize, so we need to move them around so they don't stack on top of each other."
        n121 = Unbundle By Name(w304) -> ("grid spacing"=w306:i32, "grid spacing X2"=w305:i32)
        n122 = Unbundle By Name(w304) -> ("Right Visible?"=w311:bool, "Center Visible?"=w312:bool, "Left Visible?"=w313:bool)
        n123 = property on="Left Button" class="Bool"() -> ("Position:Left"=w309:i32, "Bounds:Width"=w321:u32)  [unwired: 2 in, 2 out]
        n124 = case shown="True" w313 {
          tunnel: w309 -> [w331 w336]
          tunnel: w321 -> [_ w335]
          tunnel: [w331 w334] -> w318
          tunnel: w306 -> [_ w332]
          tunnel: [0 w332] -> w317
          frame False {
          }
          frame True {
            n125 = To Long Integer(number=w335) -> (32bit integer=w333:i32)
            n126 = Add(x=w336, y=w333) -> (x+y=w334:i32)
          }
        }
        n127 = Add(x=w318, y=w317) -> (x+y=w322:i32)
        n128 = Subtract(x=w309, y=w306) -> (x-y=w324:i32)
        n129 = case shown="True" w312 {
          tunnel: w322 -> [w346 w351]
          tunnel: [w346 w350] -> w320
          tunnel: [0 w347] -> w316
          tunnel: w306 -> [_ w347]
          frame False {
          }
          frame True {
            n130 = property on="Center Button" class="Bool"("Position:Left"=w351) -> ("Bounds:Width"=w349:u32)  [unwired: 2 in, 2 out]
            n131 = To Long Integer(number=w349) -> (32bit integer=w348:i32)
            n132 = Add(x=w348, y=w351) -> (x+y=w350:i32)
          }
        }
        n133 = Add(x=w320, y=w316) -> (x+y=w323:i32)
        n134 = case shown="True" w311 {
          tunnel: w323 -> [w338 w344]
          tunnel: [w338 w342] -> w319
          tunnel: [0 w339] -> w315
          tunnel: w306 -> [_ w339]
          frame False {
          }
          frame True {
            # "position of right edge"
            n135 = property on="Right Button" class="Bool"("Position:Left"=w344) -> ("Bounds:Width"=w341:u32)  [unwired: 2 in, 2 out]
            n136 = To Long Integer(number=w341) -> (32bit integer=w340:i32)
            n137 = Add(x=w340, y=w344) -> (x+y=w343:i32)
            n138 = To Long Integer(number=w343) -> (32bit integer=w342:i32)
          }
        }
        n139 = control-ref of="C-Message"() -> (w314:refnum<vi>)
        n140 = call <vilib>:"Longest Line Length in Pixels.vi"("String"=w314) -> ("longest line length"=w307:i32)  [unwired: 9 in]
        n141 = Add(x=w319, y=w315) -> (x+y=w325:i32)
        n142 = Add(x=w305, y=w307) -> (x+y=w326:i32)
        n143 = Subtract(x=w325, y=w324) -> (x-y=w310:i32)
        n144 = Max & Min(x=w310, y=w326) -> (max(x,y)=w308:i32)  [unwired: 1 out]
        n145 = Bundle By Name(cluster=w304, "minimum window width for buttons"=w310, "Left Button Position:Left"=w309, "mimimum window width"=w308, "minimum width for message"=w307) -> (w303:T6)
        n146 = call <vilib>:"Add State(s) to Queue__jki_lib_state_machine.vi"("State(s) in (\"\")"=w329) -> ("States Out"=w328:string)  [unwired: 14 in]
      }
      frame "UI: Resize Message Vertical" {
        w360 = u32 25  # Number of lines of text
        # "Height of one line of text (use this instead of a pre-recorded value to handle differences in font on different platforms)."
        # "This frame of the sequence takes care of resizing vertically the C-Message (the text the user sees). Normally, the string control is resized to show the entire text. But we want to bound this growth if it would make the dialog larger than the screen size. If that happens, we only grow some, and turn on the vertical scrollbar. Our arbitrary boundary for growith is a certain number of lines of text. We decided not to use screen size because some platforms, such as MS Windows, have Task Bars or similar objects that take up screen space whose size cannot be accounted for. But we assume that whatever the display, space will be available for a reasonable amount of text."
        n147 = Unbundle By Name(w353) -> ("C Message Height"=w352:u32)
        n148 = invoke on="C-Message" class="Str" method="Size to Text"() -> (error out=w354:errorcluster)  [unwired: 3 in, 2 out]
        n149 = property on="C-Message" class="Str"(error in=w354) -> (error out=w359:errorcluster, "Height"=w355:u32)  [unwired: 1 in, 1 out]
        n150 = Multiply(x=w352, y=w360) -> (x*y=w361:u32)
        n151 = Greater?(x=w355, y=w361) -> (0:w356:bool)
        n152 = case shown="False" w356 {
          selector: w356 -> [w366 w368]
          tunnel: [w365 w369] -> w357
          tunnel: [w366 w368] -> w358
          tunnel: w359 -> [w365 _]
          tunnel: w361 -> [_ w367]
          frame False {
          }
          frame True {
            n153 = property on="C-Message" class="Str"("Height"=w367) -> (error out=w369:errorcluster)  [unwired: 2 in, 1 out]
          }
        }
        n154 = property on="C-Message" class="Str"(error in=w357, "VScrollVis"=w358) -> ()  [unwired: 1 in, 2 out]
        n155 = call <vilib>:"Add State(s) to Queue__jki_lib_state_machine.vi"("State(s) in (\"\")"=w364) -> ("States Out"=w363:string)  [unwired: 14 in]
      }
      frame "UI: Resize Window to Fit Vertical" {
        # "Resize the message box to show all the text, and then VERTICALLY resize the window so scrollbars aren't necessary. (We do horizontal resize later.)"
        n156 = Unbundle By Name(w373) -> ("grid spacing"=w372:i32, "grid spacing X2"=w371:i32, "Core.Current VI Reference"=w370:refnum<vi>)
        n157 = property on="C-Message" class="Str"() -> ("Position:Top"=w389:i32, "Bounds:Height"=w390:u32)  [unwired: 2 in, 2 out]
        n158 = To Long Integer(number=w390) -> (32bit integer=w383:i32)
        n159 = Add(x=w389, y=w383) -> (x+y=w382:i32)
        n160 = Add(x=w382, y=w372) -> (x+y=w387:i32)
        n161 = property on="Left Button" class="Bool"("Position:Top"=w387) -> ("Bounds:Height"=w386:u32)  [unwired: 2 in, 2 out]
        n162 = property on="Center Button" class="Bool"("Position:Top"=w387) -> ()  [unwired: 2 in, 2 out]
        n163 = property on="Right Button" class="Bool"("Position:Top"=w387) -> ()  [unwired: 2 in, 2 out]
        n164 = property class="VI"(reference=w370) -> (reference out=w376:refnum<vi>, error out=w375:errorcluster, "Front Panel Window:Panel Bounds"=w385:T10)  [unwired: 1 in]
        n165 = To Long Integer(number=w386) -> (32bit integer=w388:i32)
        n166 = Add(x=w388, y=w387) -> (x+y=w381:i32)
        n167 = Unbundle By Name(w385) -> ("Top"=w378:i16)
        n168 = Add(x=w381, y=w371) -> (x+y=w380:i32)
        n169 = Subtract(x=w380, y=w389) -> (x-y=w377:i32)
        n170 = To Long Integer(number=w378) -> (32bit integer=w384:i32)
        n171 = Add(x=w377, y=w384) -> (x+y=w379:i32)
        n172 = Bundle By Name(cluster=w385, "Bottom"=w379) -> (w374:T10)
        n173 = property class="VI"(reference=w376, error in=w375, "Front Panel Window:Panel Bounds"=w374) -> ()  [unwired: 2 out]
        n174 = call <vilib>:"Add State(s) to Queue__jki_lib_state_machine.vi"("State(s) in (\"\")"=w393) -> ("States Out"=w392:string)  [unwired: 14 in]
      }
      frame "UI: Resize Window to Fit Horizontal" {
        # "left edge in panel coords"
        # "actual width"
        # "Resize the left and\nright components\nof the window and\nset the scroll region\nso all controls are \non screen."
        # "possible width->"
        n175 = Unbundle By Name(w396) -> ("mimimum window width"=w403:i32, "Left Button Position:Left"=w405:i32, "grid spacing"=w404:i32)
        n176 = Unbundle By Name(w396) -> ("Core.Current VI Reference"=w395:refnum<vi>)
        n177 = property class="VI"(reference=w395) -> (reference out=w394:refnum<vi>, "Front Panel Window:Panel Bounds"=w411:T10)  [unwired: 1 in, 1 out]
        n178 = property on="Pane" class="Pane"() -> ("Origin"=w406:T11)  [unwired: 2 in, 2 out]
        n179 = Unbundle By Name(w411) -> ("Right"=w413:i16, "Left"=w412:i16)
        n180 = To Long Integer(number=w413) -> (32bit integer=w407:i32)
        n181 = To Long Integer(number=w412) -> (32bit integer=w408:i32)
        n182 = Subtract(x=w405, y=w404) -> (x-y=w409:i32)
        n183 = Subtract(x=w407, y=w408) -> (x-y=w414:i32)
        n184 = Greater?(x=w403, y=w414) -> (0:w410:bool)
        n185 = case shown="False" w410 {
          tunnel: w414 -> [w419 w439]
          tunnel: w403 -> [_ w426]
          tunnel: w407 -> [_ w434]
          tunnel: w408 -> [_ w435]
          tunnel: w411 -> [_ w436]
          tunnel: [w421 w428] -> w399
          tunnel: w406 -> [w420 w429]
          tunnel: w409 -> [w421 w427]
          tunnel: [w419 w426] -> w400
          tunnel: w394 -> [_ w422]
          frame False {
            # "left edge in panel coords"
            # "actual width"
            # "Leave window width unchanged."
            n186 = Bundle By Name(cluster=w420, "Horizontal"=w421) -> (w418:T11)
            n187 = property on="Pane" class="Pane"("Origin"=w418) -> ()  [unwired: 2 in, 2 out]
          }
          frame True {
            # "left edge in panel coords"
            # "actual width"
            n188 = Subtract(x=w426, y=w439) -> (x-y=w438:i32)
            n189 = Quotient & Remainder(x=w438, y=2) -> (floor(x/y)=w431:i32)  [unwired: 1 out]
            n190 = To Long Integer(number=w431) -> (32bit integer=w425:i32)
            n191 = Subtract(x=w435, y=w425) -> (x-y=w432:i32)
            n192 = Subtract(x=w427, y=w425) -> (x-y=w428:i32)
            n193 = Add(x=w434, y=w425) -> (x+y=w433:i32)
            n194 = Bundle By Name(cluster=w429, "Horizontal"=w428) -> (w423:T11)
            n195 = Bundle By Name(cluster=w436, "Right"=w433, "Left"=w432) -> (w430:T10)
            n196 = property class="VI"(reference=w422, "Front Panel Window:Panel Bounds"=w430) -> (error out=w424:errorcluster)  [unwired: 1 in, 1 out]
            n197 = property on="Pane" class="Pane"(error in=w424, "Origin"=w423) -> ()  [unwired: 1 in, 2 out]
          }
        }
        n198 = Quotient & Remainder(x=w400, y=2) -> (floor(x/y)=w402:i32)  [unwired: 1 out]
        n199 = Add(x=w402, y=w399) -> (x+y=w398:i32)
        n200 = Bundle By Name(cluster=w396, "window center"=w398) -> (w397:T6)
        n201 = call <vilib>:"Add State(s) to Queue__jki_lib_state_machine.vi"("State(s) in (\"\")"=w417) -> ("States Out"=w416:string)  [unwired: 14 in]
      }
      frame "UI: Justify Message" {
        # "The total width of the buttons (calculated earlier) is used to figure out where the left edge of the Left Button should go and all others follow from there."
        n202 = Unbundle By Name(w448) -> ("Justify Message (Left)"=w447:enum16{"Left", "Center", "Right"}, "window center"=w446:i32, "minimum width for message"=w445:i32, "minimum window width for buttons"=w444:i32, "grid spacing X2"=w443:i32, "Left Visible?"=w442:bool, "Center Visible?"=w441:bool, "grid spacing"=w440:i32)
        n203 = Subtract(x=w444, y=w443) -> (x-y=w450:i32)
        n204 = Quotient & Remainder(x=w450, y=2) -> (floor(x/y)=w451:i32)  [unwired: 1 out]
        n205 = Quotient & Remainder(x=w445, y=2) -> (floor(x/y)=w456:i32)  [unwired: 1 out]
        n206 = Subtract(x=w446, y=w451) -> (x-y=w452:i32)
        n207 = case shown="\"Left\", Default" w447 {
          tunnel: w446 -> [w462 w468 w470]
          tunnel: w456 -> [w460 w467 _]
          frame "Left", Default {
            # "Left alignment:\n   Center point of window\n-  1/2 width of text\n------------------------------\n   Correct left position"
            n208 = Subtract(x=w462, y=w460) -> (x-y=w461:i32)
            n209 = property on="C-Message" class="Str"("Position:Left"=w461) -> ()  [unwired: 2 in, 2 out]
          }
          frame "Right" {
            # "Right alignment:\n   Center point of window\n+  1/2 width of text\n------------------------------\n   Correct right position\n-  Width of control\n-----------------------------\n   Correct left position"
            n210 = property on="C-Message" class="Str"() -> ("Bounds:Width"=w464:u32)  [unwired: 2 in, 2 out]
            n211 = Add(x=w468, y=w467) -> (x+y=w466:i32)
            n212 = To Long Integer(number=w464) -> (32bit integer=w463:i32)
            n213 = Subtract(x=w466, y=w463) -> (x-y=w465:i32)
            n214 = property on="C-Message" class="Str"("Position:Left"=w465) -> ()  [unwired: 2 in, 2 out]
          }
          frame "Center" {
            # "Center alignment:\n   Center point of window\n-  1/2 width of control\n------------------------------\n   Correct left position\n\n(the text is itself centered in the control, so centering control centers text)"
            n215 = property on="C-Message" class="Str"() -> ("Bounds:Width"=w473:u32)  [unwired: 2 in, 2 out]
            n216 = To Long Integer(number=w473) -> (32bit integer=w471:i32)
            n217 = Quotient & Remainder(x=w471, y=2) -> (floor(x/y)=w469:i32)  [unwired: 1 out]
            n218 = Subtract(x=w470, y=w469) -> (x-y=w472:i32)
            n219 = property on="C-Message" class="Str"("Position:Left"=w472) -> ()  [unwired: 2 in, 2 out]
          }
        }
        n220 = case shown="True" w442 {
          tunnel: w440 -> [_ w490]
          tunnel: w452 -> [w485 w489]
          tunnel: [w484 w487] -> w453
          frame False {
            n221 = Add(x=w485, y=0) -> (x+y=w484:i32)
          }
          frame True {
            n222 = property on="Left Button" class="Bool"("Position:Left"=w489) -> ("Bounds:Width"=w488:u32)  [unwired: 2 in, 2 out]
            n223 = To Long Integer(number=w488) -> (32bit integer=w486:i32)
            n224 = Compound Arithmetic op=ADD(w486, w489, w490) -> (w487:i32)
          }
        }
        n225 = case shown="True" w441 {
          tunnel: w440 -> [_ w482]
          tunnel: w453 -> [w477 w480]
          tunnel: [w476 w479] -> w454
          frame False {
            n226 = Add(x=w477, y=0) -> (x+y=w476:i32)
          }
          frame True {
            n227 = property on="Center Button" class="Bool"("Position:Left"=w480) -> ("Bounds:Width"=w481:u32)  [unwired: 2 in, 2 out]
            n228 = To Long Integer(number=w481) -> (32bit integer=w478:i32)
            n229 = Compound Arithmetic op=ADD(w478, w480, w482) -> (w479:i32)
          }
        }
        n230 = property on="Right Button" class="Bool"("Position:Left"=w454) -> ()  [unwired: 2 in, 2 out]
        n231 = call <vilib>:"Add State(s) to Queue__jki_lib_state_machine.vi"("State(s) in (\"\")"=w459) -> ("States Out"=w458:string)  [unwired: 14 in]
      }
      frame "UI: Assign Key Focus" {
        n232 = Unbundle By Name(w493) -> ("Left Visible?"=w492:bool, "Center Visible?"=w491:bool)
        n233 = case "Left Button Visible?" shown="True" w492 {
          tunnel: w491 -> [w501 _]
          frame False {
            n234 = control-ref of="Center Button"() -> (w500:refnum<vi>)
            n235 = control-ref of="Right Button"() -> (w499:refnum<vi>)
            n236 = Select(t=w500, s=w501, f=w499) -> (s? t:f=w498:refnum<vi>)
            n237 = property class="Bool"(reference=w498, "Key Focus"=TRUE) -> ()  [unwired: 1 in, 2 out]
          }
          frame True {
            n238 = property on="Left Button" class="Bool"("Key Focus"=TRUE) -> ()  [unwired: 2 in, 2 out]
          }
        }
        n239 = call <vilib>:"Add State(s) to Queue__jki_lib_state_machine.vi"("State(s) in (\"\")"=w496) -> ("States Out"=w495:string)  [unwired: 14 in]
      }
    }
  }
  n240 = Unbundle By Name(w3) -> ("Which Button?"=→"Which Button?":T1)
